vi "Get Spectrum.vi"(8 "error in (no error)":errorcluster, 10 "Channel":u8, 11 "Ocean Optics Driver in":refnum<class "Ocean Optics Driver.lvclass">) -> (0 "error out":errorcluster, 2 "Spectrum Graph":T1(graph), 3 "Ocean Optics Driver out":refnum<class "Ocean Optics Driver.lvclass">)   [LabVIEW 2016, in "Ocean Optics Driver.lvclass"]
uses:
  Ocean Optics Driver.lvclass
  <instrlib>/Ocean Optics 2000 4000/Ocean Optics 2000 4000.lvlib
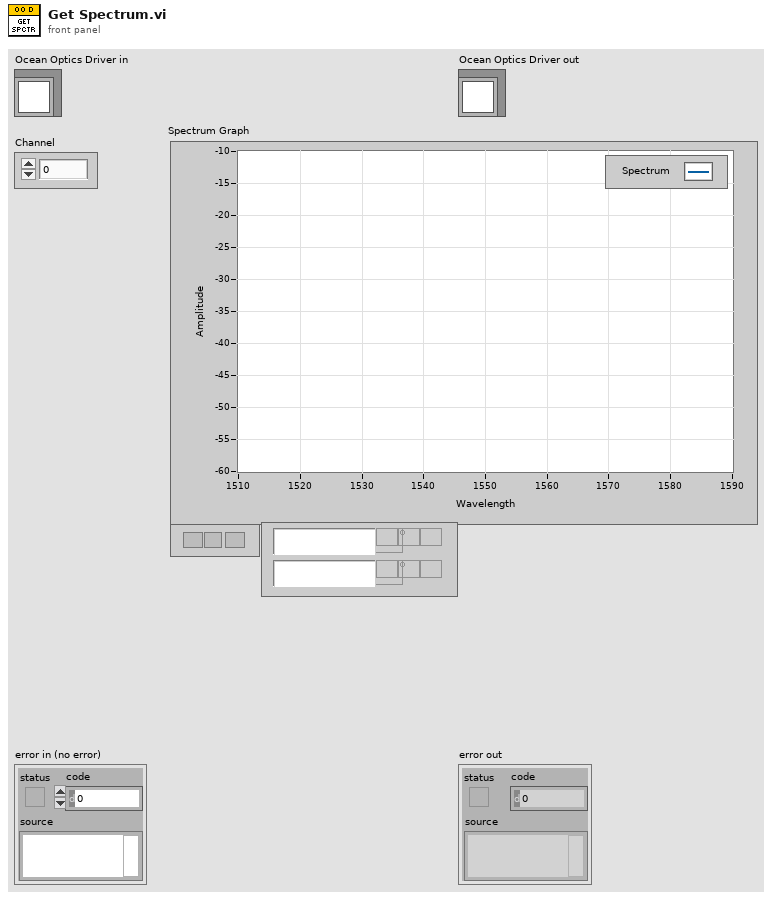
[diagram p1: front panel]
types:
  T1 = cluster{"Wavelengths":dbl[], "Spectrum by Pixel Number":dbl[]}[]
  T2 = typedef "Ruby Spectra.lvclass/Ocean optics configuration.ctl" = cluster{"Integration time":dbl, "Fit parameters":T3, "Fit":bool, "Auto-update params":bool, "Save spectra":bool, "Reference wavelengh":dbl, "Background":path}
  T3 = typedef "Multi-peak Parameters.ctl" = cluster{"Function":enum16{"Gauss", "Lorentz"}, "Window width":dbl, "Initial guess":T4}
  T4 = typedef "Peak Parameters.ctl" = cluster{"Amplitude":dbl, "Center":dbl, "Width":dbl}
  T5 = cluster{"Accessors:Wavelengths":dbl[], "Spectrum out":dbl[]}
  T6 = cluster{"Accessors:Wavelengths":dbl[], "Spectrum out":dbl[]}[]
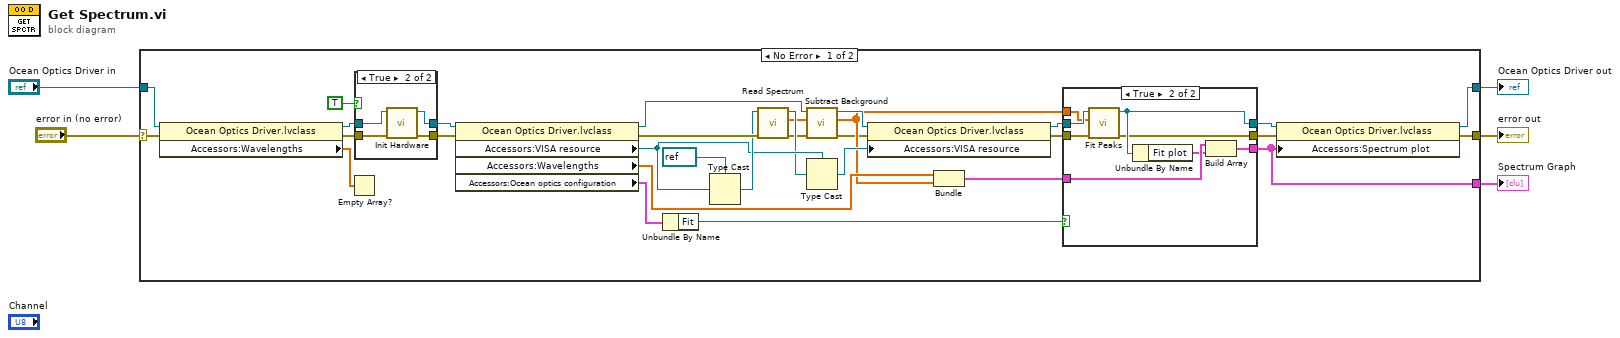
[diagram p0: block diagram]
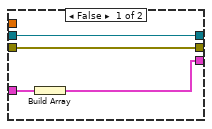
[diagram p3: hidden frame]
diagram:
  n1 = case shown="No Error" "error in (no error)" {
    selector: "error in (no error)" -> [w20 w55]
    tunnel: "Ocean Optics Driver in" -> [w18 w56]
    tunnel: [w24 w55] -> w4
    tunnel: [w22 w56] -> w3
    tunnel: [w21 _] -> w2
    frame No Error {
      n2 = property class="Ocean Optics Driver.lvclass"(reference=w18, error in=w20) -> (reference out=w16:refnum<class "Ocean Optics Driver.lvclass">, error out=w15:errorcluster, "Accessors:Wavelengths"=w17:dbl[])
      n3 = Empty Array?(array=w17) -> ()  [unwired: 1 out]
      n4 = case shown="True" TRUE {
        tunnel: w16 -> [w38 w42]
        tunnel: w15 -> [w37 w41]
        tunnel: [w38 w40] -> w14
        tunnel: [w37 w39] -> w13
        frame False {
        }
        frame True {
          n5 = call-dynamic "Init Hardware.vi"("error in (no error)"=w41, "Ocean Optics Driver in"=w42) -> ("error out"=w39:errorcluster, "Ocean Optics Driver out"=w40:refnum<class "Ocean Optics Driver.lvclass">)  [unwired: 8 in]
        }
      }
      n6 = property class="Ocean Optics Driver.lvclass"(reference=w14, error in=w13) -> (reference out=w11:refnum<class "Ocean Optics Driver.lvclass">, error out=w35:errorcluster, "Accessors:VISA resource"=w33:refnum<visa-resource-name>, "Accessors:Wavelengths"=w19:dbl[], "Accessors:Ocean optics configuration"=w30:T2)
      n7 = Unbundle By Name(w30) -> ("Fit"=w29:bool)
      n8 = Type Cast(type=refnum<visa-resource-name> refnum ("VISA resource name"), x=w33) -> (*(type *) &x=w34:refnum<visa-resource-name>)
      n9 = call <instrlib>:"Read Spectrum.vi"("error in (no error)"=w35, "VISA resource name"=w34) -> ("error out"=w9:errorcluster, "Spectrum by Pixel Number"=w8:dbl[], "VISA resource name out"=w32:refnum<visa-resource-name>)  [unwired: 6 in, 1 out]
      n10 = call-dynamic "Subtract Background.vi"("error in (no error)"=w9, "Spectrum"=w8, "Ocean Optics Driver in"=w11) -> ("error out"=w6:errorcluster, "Spectrum out"=w7:dbl[], "Ocean Optics Driver out"=w10:refnum<class "Ocean Optics Driver.lvclass">)  [unwired: 6 in]
      n11 = Type Cast(type=w33, x=w32) -> (*(type *) &x=w31:refnum<visa-resource-name>)
      n12 = property class="Ocean Optics Driver.lvclass"(reference=w10, error in=w6, "Accessors:VISA resource"=w31) -> (reference out=w28:refnum<class "Ocean Optics Driver.lvclass">, error out=w27:errorcluster)
      n13 = Bundle("Accessors:Wavelengths"=w19, "Spectrum out"=w7) -> (w25:T5)  [unwired: 1 out]
      n14 = case shown="True" w29 {
        tunnel: w28 -> [w44 w54]
        tunnel: w27 -> [w43 w53]
        tunnel: w7 -> [_ w52]
        tunnel: w25 -> [w46 w51]
        tunnel: [w45 w49] -> w21
        tunnel: [w44 w48] -> w23
        tunnel: [w43 w47] -> w26
        frame False {
          n15 = Build Array(w46) -> (w45:T6)
        }
        frame True {
          n16 = call-dynamic "Fit Peaks.vi"("error in (no error)"=w53, "Y"=w52, "Ocean Optics Driver in"=w54) -> ("error out"=w47:errorcluster, "Ocean Optics Driver out"=w48:refnum<class "Ocean Optics Driver.lvclass">)  [unwired: 7 in]
          n17 = Unbundle By Name(w48) -> ("Fit plot"=w50:cluster{"Array":dbl[], "Array":dbl[]})
          n18 = Build Array(w51, w50) -> (w49:cluster{"Array":dbl[], "Array":dbl[]}[])
        }
      }
      n19 = property class="Ocean Optics Driver.lvclass"(reference=w23, error in=w26, "Accessors:Spectrum plot"=w21) -> (reference out=w22:refnum<class "Ocean Optics Driver.lvclass">, error out=w24:errorcluster)
    }
    frame Error {
    }
  }
  "error out" <- w4
  "Ocean Optics Driver out" <- w3
  "Spectrum Graph" <- w2
